vi "Ventilador1.vi"() -> ()   [LabVIEW 2019]
uses:
  <vilib>/Analysis/polynomials.llb/Polynomial Roots (DBL).vi
  <vilib>/Analysis/NI_AALPro.lvlib
panel:
  in  "OK Button":bool
  in  "Root 3":dbl
  in  "Root 2":dbl
  in  "Root 1":dbl
  in  "Incremento":dbl
  in  "Fluxo inicial":dbl
  in  "STOP":bool=TRUE
  out "Tempos de inspirações possíveis":cdb[](array[numeric])
  out "Time":u32(graph)
  out "Signal":dbl(graph)
  in  "stop":bool
  in  "Tempo de respiração":dbl
  in  "Proporção Inspiração/respiração":string(combo)
  in  "Tempo corrido":dbl
  in  "Tipo de ventilação":string(combo)
  in  "Tipo de ciclo":string(combo)
  in  "Volume corrente":dbl
  in  "Tempo expiratório":dbl
  in  "Tempo inspiratório":dbl
  out "Fluxo respiratório medido":dbl
  in  "Frequência respiratória":dbl
  in  "Forma de onda":string(combo)
  in  "Fluxo respiratório set point":dbl
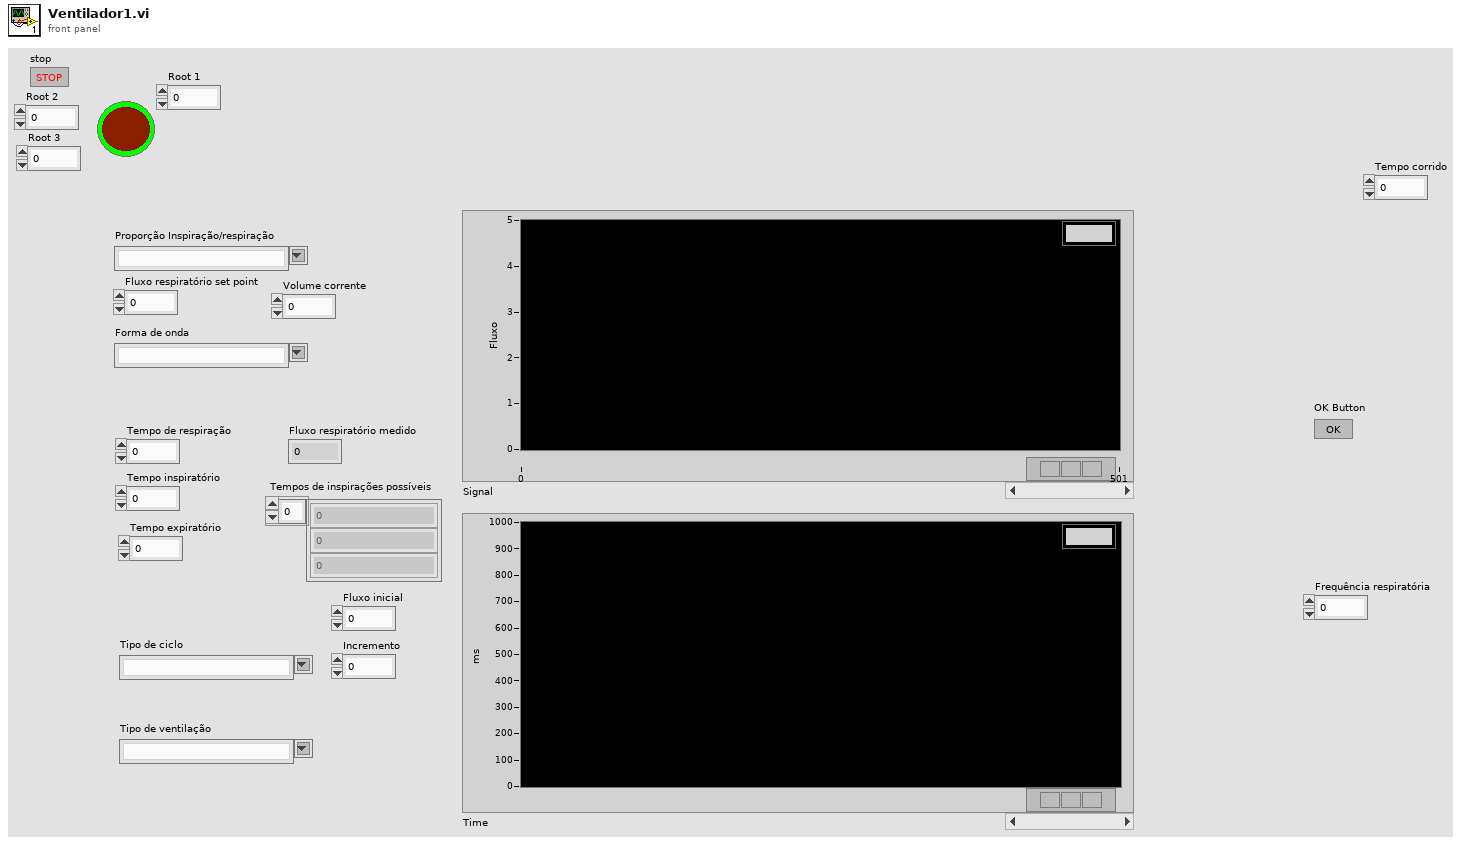
[diagram p1: front panel]
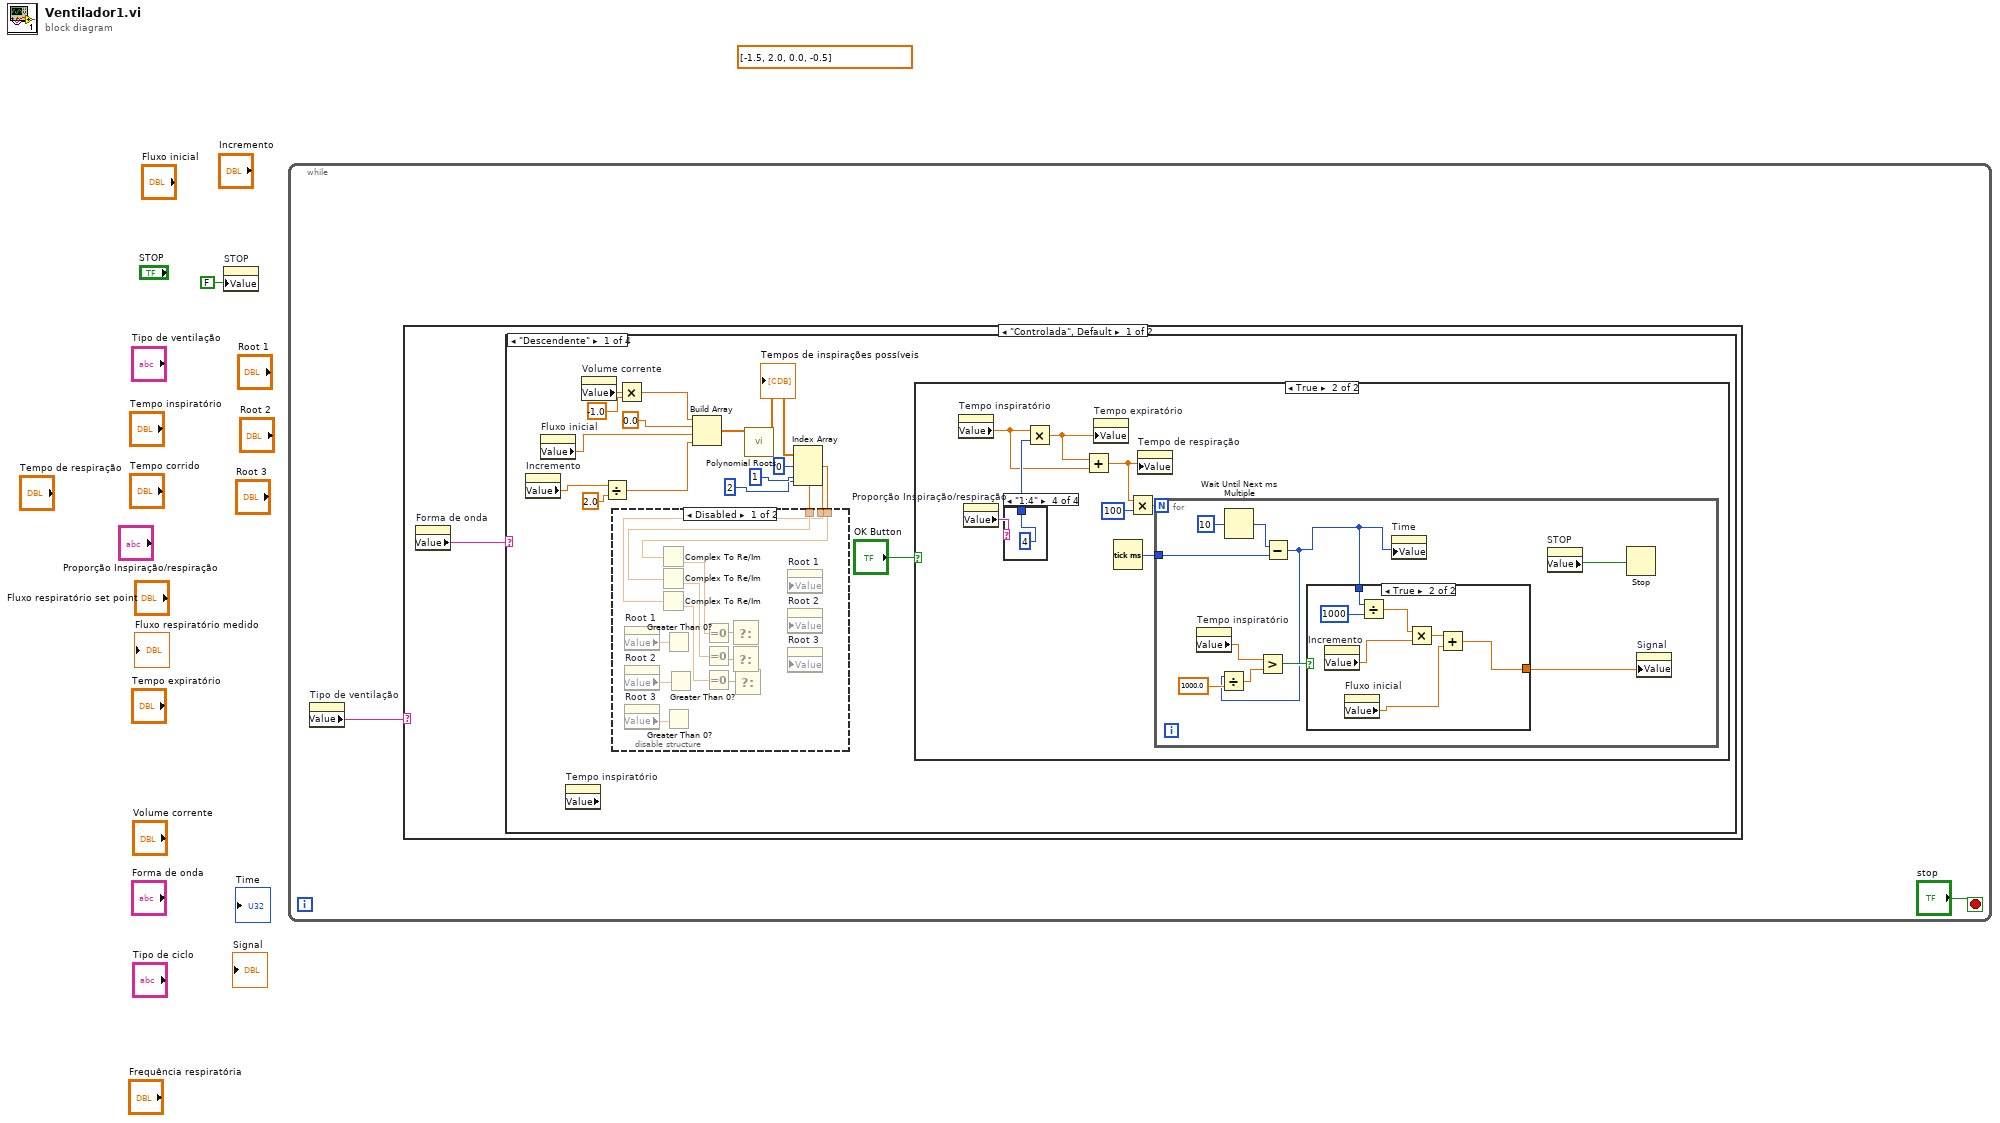
[diagram p0: block diagram]
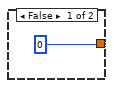
[diagram p4: hidden frame]
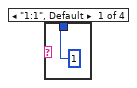
[diagram p5: hidden frame]
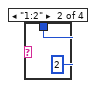
[diagram p6: hidden frame]
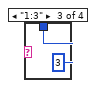
[diagram p7: hidden frame]
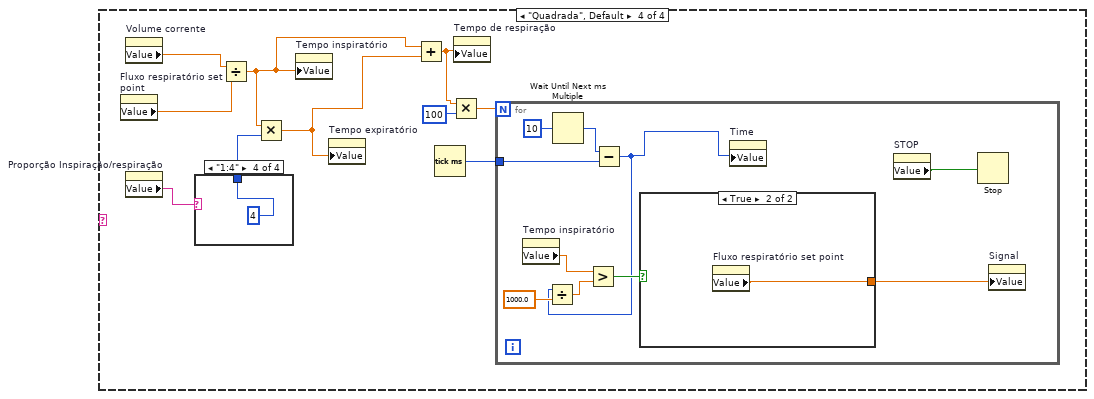
[diagram p10: hidden frame]
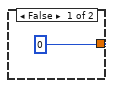
[diagram p11: hidden frame]
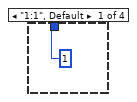
[diagram p12: hidden frame]
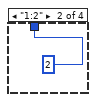
[diagram p13: hidden frame]
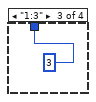
[diagram p14: hidden frame]
diagram:
  (unwired) dbl[] [-1.5, 2.0, 0.0, -0.5] ("P(x)")
  n1 = property on="STOP" class="Bool (strict)"("Value"=FALSE ("STOP")) -> ()  [unwired: 2 in, 2 out]
  n2 = while {
    stop <- "stop" stop-if-true
    n3 = property on="Tipo de ventilação" class="CmbBox"() -> ("Value"=w3:string)  [unwired: 2 in, 2 out]
    n4 = case shown="\"Controlada\", Default" w3 {
      frame "Controlada", Default {
        n5 = property on="Forma de onda" class="CmbBox"() -> ("Value"=w4:string)  [unwired: 2 in, 2 out]
        n6 = case shown="\"Descendente\"" w4 {
          frame "Descendente" {
            n7 = property on="Incremento" class="DigNum (strict)"() -> ("Value"=w20:dbl)  [unwired: 2 in, 2 out]
            n8 = property on="Fluxo inicial" class="DigNum (strict)"() -> ("Value"=w9:dbl)  [unwired: 2 in, 2 out]
            n9 = property on="Tempo inspiratório" class="DigNum (strict)" props=["Value"]() -> ()  [unwired: 2 in, 3 out]
            n10 = property on="Volume corrente" class="DigNum (strict)"() -> ("Value"=w19:dbl)  [unwired: 2 in, 2 out]
            n11 = Divide(x=w20, y=2.0) -> (x/y=w8:dbl)
            n12 = Multiply(x=w19, y=-1.0) -> (x*y=w11:dbl)
            n13 = Build Array(w11, 0.0 ("element"), w9, w8) -> (w7:dbl[])
            n14 = call-poly <vilib>:"Polynomial Roots.vi"("P(x)"=w7) -> ("Roots"=w21:cdb[])  [unwired: 9 in, 1 out]
            "Tempos de inspirações possíveis" <- w21
            n15 = Index Array(array=w21, index #1=0 ("index"), index #2=1 ("index"), index #3=2 ("index")) -> (element #1=w6:cdb, element #2=w13:cdb, element #3=w12:cdb)
            n16 = disable-structure shown="Disabled" {
              disable-tunnel: w13 -> [w33 _]
              disable-tunnel: w12 -> [w32 _]
              disable-tunnel: w6 -> [w31 _]
              frame Disabled {
                n17 = property on="Root 1" class="DigNum (strict)"() -> ("Value"=w30:dbl)  [unwired: 2 in, 2 out]
                n18 = property on="Root 2" class="DigNum (strict)"() -> ("Value"=w29:dbl)  [unwired: 2 in, 2 out]
                n19 = property on="Root 3" class="DigNum (strict)"() -> ("Value"=w28:dbl)  [unwired: 2 in, 2 out]
                n20 = Complex To Re/Im(x + iy=w31) -> (y=w25:dbl)  [unwired: 1 out]
                n21 = Complex To Re/Im(x + iy=w33) -> (y=w26:dbl)  [unwired: 1 out]
                n22 = Complex To Re/Im(x + iy=w32) -> (y=w27:dbl)  [unwired: 1 out]
                n23 = Greater Than 0?(x=w30) -> ()  [unwired: 1 out]
                n24 = Greater Than 0?(x=w28) -> ()  [unwired: 1 out]
                n25 = Greater Than 0?(x=w29) -> ()  [unwired: 1 out]
                n26 = Equal To 0?(x=w25) -> (x = 0?=w24:bool)
                n27 = Equal To 0?(x=w26) -> (x = 0?=w23:bool)
                n28 = Equal To 0?(x=w27) -> (x = 0?=w22:bool)
                n29 = Select(s=w24) -> ()  [unwired: 2 in, 1 out]
                n30 = Select(s=w23) -> ()  [unwired: 2 in, 1 out]
                n31 = Select(s=w22) -> ()  [unwired: 2 in, 1 out]
                n32 = property on="Root 1" class="DigNum (strict)" props=["Value"]() -> ()  [unwired: 3 in, 2 out]
                n33 = property on="Root 2" class="DigNum (strict)" props=["Value"]() -> ()  [unwired: 3 in, 2 out]
                n34 = property on="Root 3" class="DigNum (strict)" props=["Value"]() -> ()  [unwired: 3 in, 2 out]
              }
              frame Enabled {
              }
            }
            n35 = case shown="True" "OK Button" {
              frame False {
              }
              frame True {
                n36 = property on="Tempo inspiratório" class="DigNum (strict)"() -> ("Value"=w35:dbl)  [unwired: 2 in, 2 out]
                n37 = property on="Proporção Inspiração/respiração" class="CmbBox"() -> ("Value"=w41:string)  [unwired: 2 in, 2 out]
                n38 = case shown="\"1:4\"" w41 {
                  tunnel: [1 2 3 4] -> w37
                  frame "1:1", Default {
                  }
                  frame "1:2" {
                  }
                  frame "1:3" {
                  }
                  frame "1:4" {
                  }
                }
                n39 = Multiply(x=w35, y=w37) -> (x*y=w36:dbl)
                n40 = Add(x=w36, y=w35) -> (x+y=w34:dbl)
                n41 = property on="Tempo expiratório" class="DigNum (strict)"("Value"=w36) -> ()  [unwired: 2 in, 2 out]
                n42 = Tick Count (ms)() -> (millisecond timer value=w40:u32)
                n43 = Multiply(x=w34, y=100) -> (x*y=w39:dbl)
                n44 = property on="Tempo de respiração" class="DigNum (strict)"("Value"=w34) -> ()  [unwired: 2 in, 2 out]
                n45 = for {
                  N: w39 -> [_]
                  tunnel: w40 -> [w49]
                  n46 = property on="Tempo inspiratório" class="DigNum (strict)"() -> ("Value"=w47:dbl)  [unwired: 2 in, 2 out]
                  n47 = Wait Until Next ms Multiple(millisecond multiple=u32 10) -> (millisecond timer value=w51:u32)
                  n48 = Subtract(x=w51, y=w49) -> (x-y=w43:u32)
                  n49 = Divide(x=w43, y=1000.0) -> (x/y=w46:dbl)
                  n50 = Greater?(x=w47, y=w46) -> (0:w48:bool)
                  n51 = case shown="True" w48 {
                    tunnel: [0 w54] -> w42
                    tunnel: w43 -> [_ w59]
                    frame False {
                    }
                    frame True {
                      n52 = property on="Incremento" class="DigNum (strict)"() -> ("Value"=w56:dbl)  [unwired: 2 in, 2 out]
                      n53 = property on="Fluxo inicial" class="DigNum (strict)"() -> ("Value"=w53:dbl)  [unwired: 2 in, 2 out]
                      n54 = Divide(x=w59, y=u32 1000) -> (x/y=w57:dbl)
                      n55 = Multiply(x=w57, y=w56) -> (x*y=w55:dbl)
                      n56 = Add(x=w55, y=w53) -> (x+y=w54:dbl)
                    }
                  }
                  n57 = property on="Time" class="WFChart (strict)"("Value"=w43) -> ()  [unwired: 2 in, 2 out]
                  n58 = property on="STOP" class="Bool (strict)"() -> ("Value"=w44:bool)  [unwired: 2 in, 2 out]
                  n59 = Stop(stop? (T)=w44) -> ()
                  n60 = property on="Signal" class="WFChart (strict)"("Value"=w42) -> ()  [unwired: 2 in, 2 out]
                }
              }
            }
          }
          frame "Ascendente" {
          }
          frame "Sinusoidal" {
          }
          frame "Quadrada", Default {
            n61 = property on="Fluxo respiratório set point" class="DigNum (strict)"() -> ("Value"=w73:dbl)  [unwired: 2 in, 2 out]
            n62 = property on="Volume corrente" class="DigNum (strict)"() -> ("Value"=w72:dbl)  [unwired: 2 in, 2 out]
            n63 = property on="Proporção Inspiração/respiração" class="CmbBox"() -> ("Value"=w71:string)  [unwired: 2 in, 2 out]
            n64 = case shown="\"1:4\"" w71 {
              tunnel: [1 2 3 4] -> w70
              frame "1:1", Default {
              }
              frame "1:2" {
              }
              frame "1:3" {
              }
              frame "1:4" {
              }
            }
            n65 = Divide(x=w72, y=w73) -> (x/y=w66:dbl)
            n66 = Multiply(x=w66, y=w70) -> (x*y=w65:dbl)
            n67 = property on="Tempo inspiratório" class="DigNum (strict)"("Value"=w66) -> ()  [unwired: 2 in, 2 out]
            n68 = property on="Tempo expiratório" class="DigNum (strict)"("Value"=w65) -> ()  [unwired: 2 in, 2 out]
            n69 = Add(x=w66, y=w65) -> (x+y=w64:dbl)
            n70 = Tick Count (ms)() -> (millisecond timer value=w69:u32)
            n71 = Multiply(x=w64, y=100) -> (x*y=w68:dbl)
            n72 = property on="Tempo de respiração" class="DigNum (strict)"("Value"=w64) -> ()  [unwired: 2 in, 2 out]
            n73 = for {
              N: w68 -> [_]
              tunnel: w69 -> [w81]
              n74 = property on="Tempo inspiratório" class="DigNum (strict)"() -> ("Value"=w79:dbl)  [unwired: 2 in, 2 out]
              n75 = Wait Until Next ms Multiple(millisecond multiple=u32 10) -> (millisecond timer value=w83:u32)
              n76 = Subtract(x=w83, y=w81) -> (x-y=w76:u32)
              n77 = Divide(x=w76, y=1000.0) -> (x/y=w78:dbl)
              n78 = Greater?(x=w79, y=w78) -> (0:w80:bool)
              n79 = case shown="True" w80 {
                tunnel: [0 w85] -> w75
                frame False {
                }
                frame True {
                  n80 = property on="Fluxo respiratório set point" class="DigNum (strict)"() -> ("Value"=w85:dbl)  [unwired: 2 in, 2 out]
                }
              }
              n81 = property on="Time" class="WFChart (strict)"("Value"=w76) -> ()  [unwired: 2 in, 2 out]
              n82 = property on="STOP" class="Bool (strict)"() -> ("Value"=w74:bool)  [unwired: 2 in, 2 out]
              n83 = Stop(stop? (T)=w74) -> ()
              n84 = property on="Signal" class="WFChart (strict)"("Value"=w75) -> ()  [unwired: 2 in, 2 out]
            }
          }
        }
      }
      frame "Expontânea/Assistida" {
      }
    }
  }
